vi "U64toRgba_1D.vi"(11 "U64":u64[](array[numeric])) -> (3 "Rgba":T1[](array[typedef]))   [LabVIEW 2024, in "OpenLvVision_Image.lvlib" / "DataAccess.lvlib"]
doc: "Convert an number into an cluster"
uses:
  DataAccess.lvlib
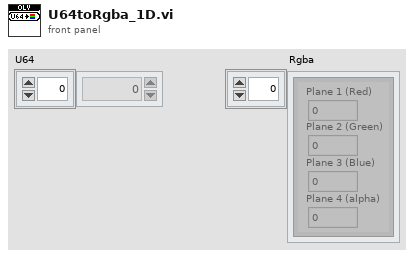
[diagram p1: front panel]
types:
  T1 = typedef "Color (U64)" = cluster{"Plane 3 (Blue)":u16, "Plane 2 (Green)":u16, "Plane 1 (Red)":u16, "Plane 4 (alpha)":u16}
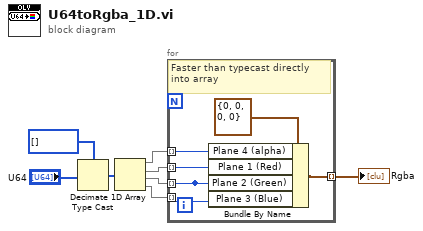
[diagram p0: block diagram]
diagram:
  n1 = Type Cast(type=u16[] [], x="U64") -> (*(type *) &x=w6:u16[])
  n2 = Decimate 1D Array(w6) -> (w5:u16[], w3:u16[], w2:u16[], w4:u16[])
  n3 = for {
    tunnel: w5 -> [w14] mode=indexing
    tunnel: w3 -> [w13] mode=indexing
    tunnel: [w10] -> _ mode=indexing
    tunnel: w4 -> [w12] mode=indexing
    tunnel: [w11] -> w1 mode=indexing
    tunnel: w2 -> [w10] mode=indexing
    # "Faster than typecast directly into array"
    n4 = Bundle By Name(cluster=T1 {"Plane 3 (Blue)"=0, "Plane 2 (Green)"=0, "Plane 1 (Red)"=0, "Plane 4 (alpha)"=0} ("Rgba"), "Plane 4 (alpha)"=w14, "Plane 1 (Red)"=w13, "Plane 2 (Green)"=w10, "Plane 3 (Blue)"=w12) -> (w11:T1)
  }
  "Rgba" <- w1
